vi "Defer Application Panel Updates.vi"(8 "error in (no error)":errorcluster, 10 "Defer Panel Updates":bool=TRUE, 11 "Application in":refnum<class "Application.lvclass">) -> (0 "error out":errorcluster, 3 "Application out":refnum<class "Application.lvclass">)   [LabVIEW 2017, in "Application.lvlib" / "Application.lvclass"]
doc: "Controls deferring of updates for the front panel of the application."
uses:
  Application.lvclass
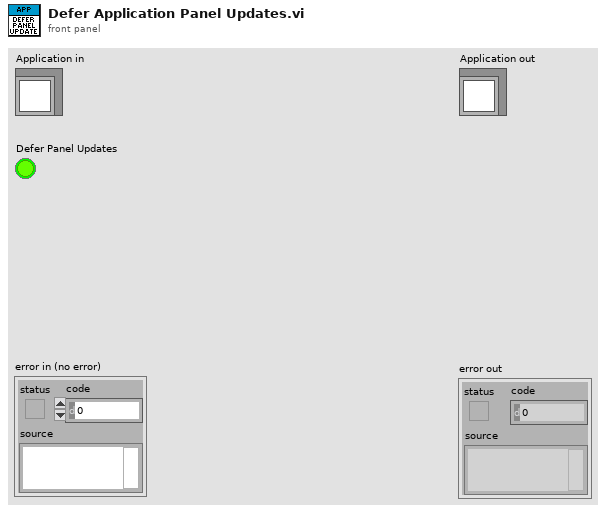
[diagram p1: front panel]
types:
  T1 = typedef "Application.lvlib/App Properties.lvclass/Class Properties -- Cluster.ctl" = cluster{"UUT Info":T2[], "Test Information":refnum<vi>, "Gold Board":refnum<class "Golden Board.lvclass">, "Test Recipe":refnum<class "Test Recipe.lvclass">, "Instruments":refnum<class "Instrument.lvclass">[], "Mode":T3, "Test Results":T4[], "Station Config":refnum<class "Station Config.lvclass">, "Variable Engine":refnum<class "Variable Engine.lvclass">}
  T2 = typedef "Application.lvlib/App Properties.lvclass/UUT Reference -- Cluster.ctl" = cluster{"Serial Number Reference":refnum<vi>, "Status Message Reference":refnum<vi>}
  T3 = typedef "Application.lvlib/Application.lvclass/Op Mode -- Enum.ctl" = u16
  T4 = typedef "Application.lvlib/App Properties.lvclass/Test Result -- Cluster.ctl" = cluster{"Position":i32, "Pass":bool, "Fail Codes":string}
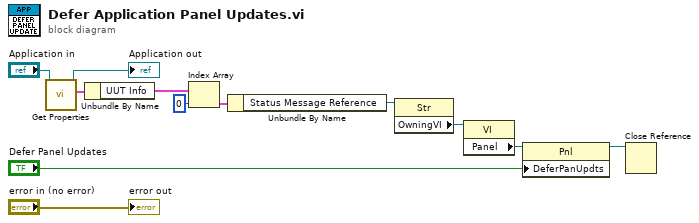
[diagram p0: block diagram]
diagram:
  n1 = call "Get Properties.vi"("Acrobat Template in"="Application in") -> ("Class Properties"=w9:T1, "Acrobat Template out"=→"Application out":refnum<class "Application.lvclass">)  [unwired: 8 in, 1 out]
  n2 = Unbundle By Name(w9) -> ("UUT Info"=w2:T2[])
  n3 = Index Array(array=w2, index=0) -> (element=w3:T2)
  n4 = Unbundle By Name(w3) -> ("Status Message Reference"=w7:refnum<vi>)
  n5 = property class="Str"(reference=w7) -> ("OwningVI"=w6:refnum<vi>)  [unwired: 1 in, 2 out]
  n6 = property class="VI"(reference=w6) -> ("Panel"=w5:refnum<vi>)  [unwired: 1 in, 2 out]
  n7 = property class="Pnl"(reference=w5, "DeferPanUpdts"="Defer Panel Updates") -> (reference out=w1:refnum<vi>)  [unwired: 1 in, 1 out]
  n8 = Close Reference(reference=w1) -> ()  [unwired: 1 in, 1 out]
  "error out" <- "error in (no error)"
